vi "PH_Beckhoff_Common.get PSDB Information for former classes.vi"(1 "PSDB Classes":T2) -> (0 "PSDB Information":T1)   [LabVIEW 2014, in "PH_Beckhoff_Common.lvlib"]
doc: "This VI creates Tagnames to be used for PSDB communication; it replaces instance- and classname of the removed classes."
uses:
  PH_Beckhoff_Common.lvlib
  PH_Beckhoff_Common.former PSDB classes.ctl
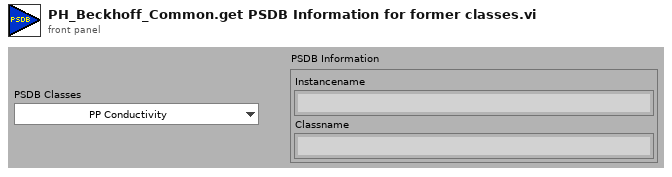
[diagram p1: front panel]
types:
  T1 = cluster{"Instancename":string, "Classname":string}
  T2 = typedef "PH_Beckhoff_Common.lvlib/PH_Beckhoff_Common.former PSDB classes.ctl" = enum16{"PP Conductivity", "PP Mercury", "PA Chiller"}
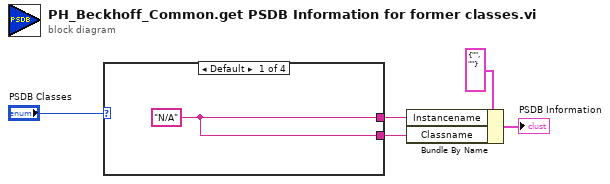
[diagram p0: block diagram]
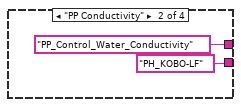
[diagram p2: hidden frame]
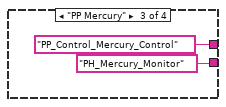
[diagram p3: hidden frame]
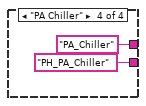
[diagram p4: hidden frame]
diagram:
  n1 = case shown="Default" "PSDB Classes" {
    tunnel: [w6 "PP_Control_Water_Conductivity" "PP_Control_Mercury_Control" "PA_Chiller"] -> w2
    tunnel: [w6 "PH_KOBO-LF" "PH_Mercury_Monitor" "PH_PA_Chiller"] -> w1
    frame Default {
      w6 = "N/A"
    }
    frame "PP Conductivity" {
    }
    frame "PP Mercury" {
    }
    frame "PA Chiller" {
    }
  }
  n2 = Bundle By Name(cluster=T1 {"Instancename"="", "Classname"=""} ("PSDB Information"), "Instancename"=w2, "Classname"=w1) -> (→"PSDB Information":T1)
